vi "rotate.vi"(8 "error in (no error)":errorcluster, 10 "angle":dbl[unit], 11 "GenericTrajectory in":refnum<class "TrajectoryDL091126GenericVoxel.lvclass">) -> (0 "error out":errorcluster, 3 "GenericTrajectory out":refnum<class "TrajectoryDL091126GenericVoxel.lvclass">)   [LabVIEW 2010, in "TrajectoryDL091126GenericVoxel.lvclass"]
uses:
  TrajectoryDL091126GenericVoxel.lvclass
  common/legacy/axes.ctl
  TrajectoryDL091126GenericVoxel.lvclass/TrajectoryDL091126GenericVoxel.ctl
  common/classes/ErrorController/ErrorController/class_data.vi
  common/classes/ErrorController/ErrorController/ErrorController.lvclass
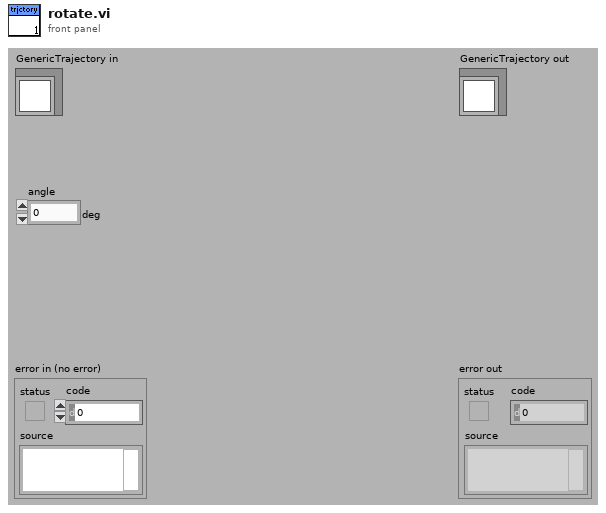
[diagram p1: front panel]
types:
  T1 = typedef "axes.ctl" = enum16{"x", "y", "z"}
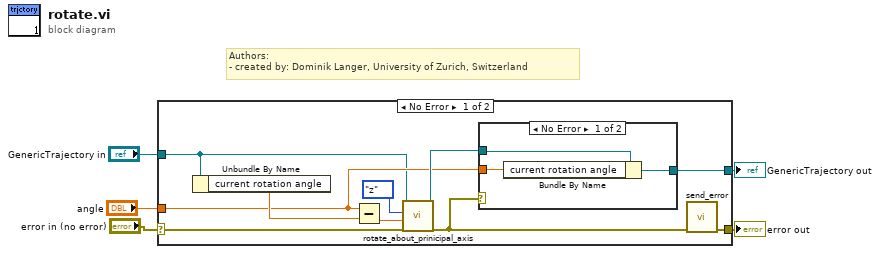
[diagram p0: block diagram]
diagram:
  # "Authors: \n- created by: Dominik Langer, University of Zurich, Switzerland"
  n1 = case shown="No Error" "error in (no error)" {
    selector: "error in (no error)" -> [w12 w21]
    tunnel: [w6 w21] -> w4
    tunnel: [w10 w20] -> w1
    tunnel: "GenericTrajectory in" -> [w8 w20]
    tunnel: "angle" -> [w9 _]
    frame No Error {
      n2 = Unbundle By Name(w8) -> ("current rotation angle"=w14:dbl[unit])
      n3 = Subtract(x=w9, y=w14) -> (x-y=w13:dbl[unit])
      n4 = call-dynamic "rotate_about_prinicipal_axis.vi"("error in (no error)"=w12, "angle"=w13, "axis"=axes."z", "GenericTrajectory in"=w8) -> ("error out"=w7:errorcluster, "GenericTrajectory out"=w11:refnum<class "TrajectoryDL091126GenericVoxel.lvclass">)  [unwired: 1 in, 5 out]
      n5 = case shown="No Error" w7 {
        tunnel: w11 -> [w18 w19]
        tunnel: [w17 w19] -> w10
        tunnel: w9 -> [w16 _]
        frame No Error {
          n6 = Bundle By Name(cluster=w18, "current rotation angle"=w16) -> (w17:refnum<class "TrajectoryDL091126GenericVoxel.lvclass">)
        }
        frame Error {
        }
      }
      n7 = call "send_error.vi"("error in (no error)"=w7) -> ("error out"=w6:errorcluster)  [unwired: 10 in]
    }
    frame Error {
    }
  }
  "error out" <- w4
  "GenericTrajectory out" <- w1
